vi "UDP_Read.vi"() -> ()   [LabVIEW 2014]
doc: "This example VI is to be used in conjunction with the UDP_Write.vi example. \nMake sure to run this example VI prior to running the UDP_Write.vi, otherwise an error will be generated. \n\nBoth the UDP_Wite.vi and UDP_Read.vi can run deployed on the Raspberry Pi; the UDP_Wite.vi can run deployed on the Raspberry Pi and the UDP_Read.vi remotely on a different networked computer or Raspberry Pi; or the UDP_Wite.vi can run remoterly on a different networked computer or Raspberry Pi and the UDP_Read.vi deployed in the Raspberry Pi target.\n\nIf both UDP_Wite.vi and UDP_Read.vi run deployed at the same Raspberry Pi, the address control value is to be left unchanged of its default 127.0.0.1 value. If the UDP_Wite.vi runs on a different computer than the UDP_Read.vi, enter the IP address of the computer running the UDP_Read.vi example in the UDP_Wite.vi remote address control.\n\nMake sure the value of the remote port control of UDP_Wite.vi matches with the local port value of the UDP_Read.vi.\n\nEnter a string message in the data in control and run the UDP_Wite.vi. Note on the running UDP_Read.vi that the remote address indicator will show the IP address of the computer where UDP_Wite.vi ran. The data out indicator of UDP_Read.vi will show the same string value entered in the UDP_Wite.vi data in control.\n\nTo stop the UDP_Read.vi execution, enter stop in the data in control and run UDP_Wite.vi."
panel:
  out "remote port":u16
  in  "error in":errorcluster
  out "error out":errorcluster
  out "remote address":string
  in  "local port":u16=6345
  out "data out":string
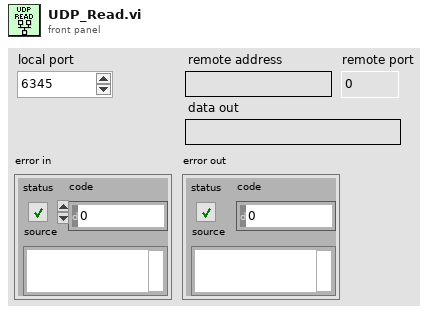
[diagram p1: front panel]
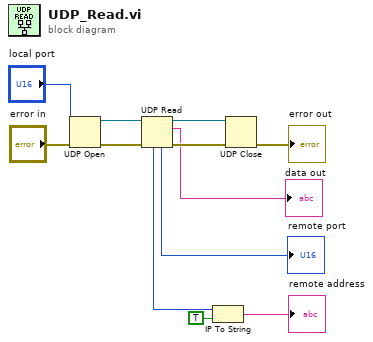
[diagram p0: block diagram]
diagram:
  n1 = UDP Open(8:"error in", 11:"local port") -> (port=w12:refnum<k16>, 0:w10:errorcluster)  [unwired: 3 in, 1 out]
  n2 = UDP Read(connection ID=w12, 8:w10) -> (data out=→"data out":string, error out=w9:errorcluster, 3:w11:refnum<k16>, 4:→"remote port":u16, 6:w3:u32)  [unwired: 2 in]
  n3 = IP To String(1:TRUE ("dot notation? (F)"), 2:w3) -> (0:→"remote address":string)
  n4 = UDP Close(connection ID=w11, 8:w9) -> (error out=→"error out":errorcluster)  [unwired: 1 out]
